vi "upload-session.vi"(4 "chunk_size_bytes":i64=157286400, 6 "timeout_ms":i32=10000, 8 "error in (no error)":errorcluster, 9 "file":string, 10 "path":string, 11 "filepath":path) -> (0 "error out":errorcluster)   [LabVIEW 2015, in "lv-dropbox.lvlib" / "v2.lvlib"]
uses:
  v2.lvlib
  lv-dropbox.lvlib
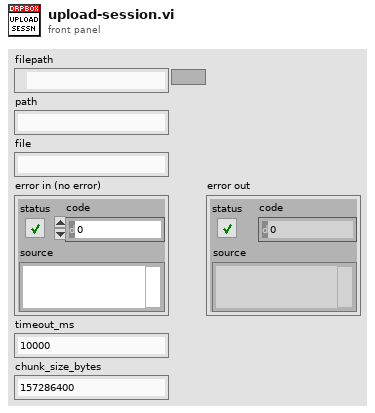
[diagram p1: front panel]
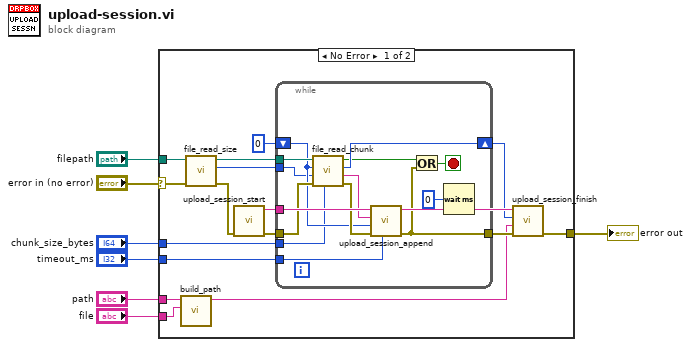
[diagram p0: block diagram]
diagram:
  n1 = case shown="No Error" "error in (no error)" {
    selector: "error in (no error)" -> [w21 w37]
    tunnel: "filepath" -> [w12 _]
    tunnel: "timeout_ms" -> [w16 _]
    tunnel: "path" -> [w10 _]
    tunnel: [w13 w37] -> w3
    tunnel: "chunk_size_bytes" -> [w11 _]
    tunnel: "file" -> [w8 _]
    frame No Error {
      n2 = call "build_path.vi"("path"=w8, "base_path"=w10) -> ("path"=w9:string)  [unwired: 9 in]
      n3 = call "file_read_size.vi"("error in (no error)"=w21, "filepath"=w12) -> ("error out"=w22:errorcluster, "size_bytes"=w17:i64)  [unwired: 8 in]
      n4 = call "upload_session_start.vi"("error in (no error)"=w22) -> ("error out"=w18:errorcluster, "session_id"=w19:string)  [unwired: 9 in]
      n5 = while {
        shift-right: [w28] -> w14
        shift-left: i64 0 -> [w27]
        tunnel: w19 -> [w33]
        tunnel: w17 -> [w24]
        tunnel: w16 -> [w32]
        tunnel: w12 -> [w29]
        tunnel: w11 -> [w25]
        tunnel: w18 -> [w36]
        tunnel: [w31] -> w15
        stop <- w30 stop-if-true
        n6 = call "file_read_chunk.vi"("chunk_size_bytes"=w25, "error in (no error)"=w36, "file_size"=w24, "offset_in"=w27, "filepath"=w29) -> ("error out"=w35:errorcluster, "data"=w34:string, "offset_out"=w28:i64, "last_chunk"=w23:bool)  [unwired: 3 in]
        n7 = call "upload_session_append.vi"("timeout_ms"=w32, "error in (no error)"=w35, "offset"=w27, "data"=w34, "session_id"=w33) -> ("error out"=w31:errorcluster)  [unwired: 6 in]
        n8 = Or(x=w23, y=w31) -> (x .or. y?=w30:bool)
        n9 = Wait (ms)(milliseconds to wait=u32 0) -> ()  [unwired: 1 out]
      }
      n10 = call "upload_session_finish.vi"("error in (no error)"=w15, "path"=w9, "offset"=w14, "session_id"=w19) -> ("error out"=w13:errorcluster)  [unwired: 7 in]
    }
    frame Error {
    }
  }
  "error out" <- w3
